vi "fromInternalIndex.vi"(1 "Internal index":u8) -> (0 "Square":T1={"File"=enum."d", "Rank"=enum."4"})   [LabVIEW 2015, in "Chesslib.lvlib" / "Board.lvclass"]
uses:
  Board.lvclass
  typedef/Square.ctl
  typedef/File.ctl
  typedef/Rank.ctl
  Chesslib.lvlib
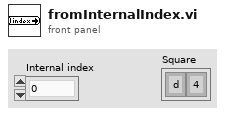
[diagram p1: front panel]
types:
  T1 = typedef "Chesslib.lvlib/Square.ctl" = cluster{"File":T2, "Rank":T3}
  T2 = typedef "Chesslib.lvlib/File.ctl" = enum8{"a", "b", "c", "d", "e", "f", "g", "h"}
  T3 = typedef "Chesslib.lvlib/Rank.ctl" = enum8{"1", "2", "3", "4", "5", "6", "7", "8"}
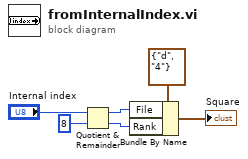
[diagram p0: block diagram]
diagram:
  n1 = Quotient & Remainder(x="Internal index", y=u8 8) -> (x-y*floor(x/y)=w2:u8, floor(x/y)=w1:u8)
  n2 = Bundle By Name(cluster=T1 {"File"=enum."d", "Rank"=enum."4"} ("Square"), "File"=w2, "Rank"=w1) -> (→"Square":T1)
